vi "Demo_Scale Analog.vi"(4 "COUNT_MIN":dbl=-32767.0, 5 "DISP_MIN":dbl=-10.0, 6 "COUNT_MAX":dbl=32767.0, 7 "DISP_MAX":dbl=10.0, 11 "Analog IN":dbl) -> (3 "Calibration OUT":dbl)   [LabVIEW 2017]
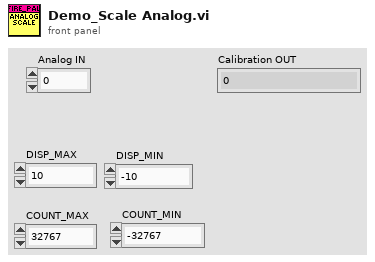
[diagram p1: front panel]
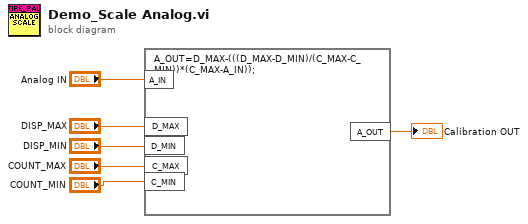
[diagram p0: block diagram]
diagram:
  n1 = formula code="A_OUT=D_MAX-(((D_MAX-D_MIN)/(C_MAX-C_MIN))*(C_MAX-A_IN));"("A_IN"="Analog IN", "D_MAX"="DISP_MAX", "D_MIN"="DISP_MIN", "C_MAX"="COUNT_MAX", "C_MIN"="COUNT_MIN") -> ("A_OUT"=→"Calibration OUT":dbl)
